vi "Check Design Array Full_2.vi"(11 "Design Data":T1) -> (3 "Design Array Full":bool)   [LabVIEW 2024]
uses:
  Cluster_Design Data_2.ctl
  ENUM_Stripe Select.ctl
  Cluster_Design Towel ID Data_2.ctl
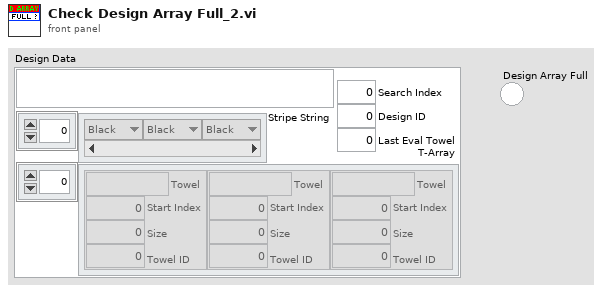
[diagram p1: front panel]
types:
  T1 = typedef "Cluster_Design Data_2.ctl" = cluster{"Stripe String":string, "Stripes":T2[], "T-Array":T3[], "Search Index":i32, "Design ID":i32, "Last Eval Towel":i32}
  T2 = typedef "ENUM_Stripe Select.ctl" = enum16{"Black", "Blue", "Green", "Red", "White"}
  T3 = typedef "Cluster_Design Towel ID Data_2.ctl" = cluster{"Towel":string, "Start Index":i32, "Size":i32, "Towel ID":i32}
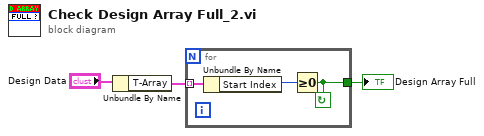
[diagram p0: block diagram]
diagram:
  n1 = Unbundle By Name("Design Data") -> ("T-Array"=w1:T3[])
  n2 = for {
    tunnel: w1 -> [w6] mode=indexing
    tunnel: [w4] -> w3
    stop <- w4 continue-if-true
    n3 = Unbundle By Name(w6) -> ("Start Index"=w5:i32)
    n4 = Greater Or Equal To 0?(x=w5) -> (x >= 0?=w4:bool)
  }
  "Design Array Full" <- w3
